vi "1) Single Group.vi"() -> ()   [LabVIEW 2020, in "VectoScratch.lvlib"]
uses:
  VectoScratch.lvlib
  Vecto/Group Info.ctl
  Vecto/Group Data Type.ctl
  Vecto/Channel Init.ctl
  Vecto/Group DBL/Group DBL.lvclass
  C:/dev/lv20CE/relink/lv-vecto/Vecto/Group/Group.lvclass
  Vecto/ChannelService/Create Group Abstract.vi
  Vecto/ChannelService/ChannelService.lvclass
  VectoConfig/VectoConfig.lvlib
  Vecto/Group Config/Group Config.lvclass
  Vecto/Group/Group.lvclass
panel:
  out "Channels":cluster{"Name":string, "Scaled":dbl}[](array[cluster])
  in  "stop":bool
  in  "Source Data":dbl[](array[slide])=[0.0, 0.0, 0.0, 0.0, 0.0] scale=0.0..10.0
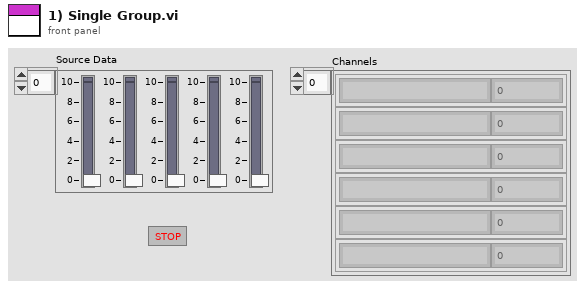
[diagram p1: front panel]
types:
  T1 = typedef "VectoConfig.lvlib/Group Data Type.ctl" = enum16{"Double", "String"}
  T2 = typedef "VectoConfig.lvlib/Group Info.ctl" = cluster{"System":string, "Cluster":string, "Node":string, "Task":string, "Name":string}
  T3 = typedef "VectoConfig.lvlib/Channel Init.ctl" = cluster{"Name":string, "Resource":string, "Unit String":string}
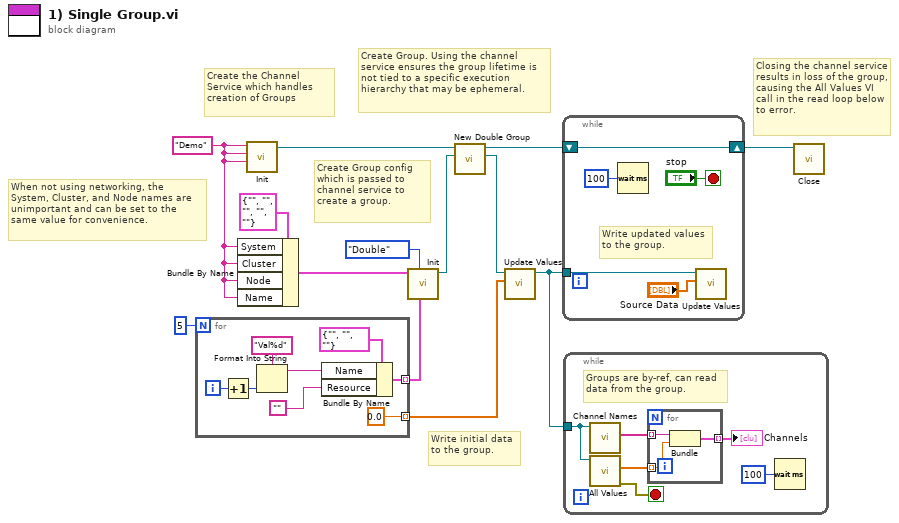
[diagram p0: block diagram]
diagram:
  w1 = "Demo" ("System")
  # "When not using networking, the System, Cluster, and Node names are unimportant and can be set to the same value for convenience."
  # "Closing the channel service results in loss of the group, causing the All Values VI call in the read loop below to error."
  # "Write initial data to the group."
  # "Create Group. Using the channel service ensures the group lifetime is not tied to a specific execution hierarchy that may be ephemeral."
  # "Create Group config which is passed to channel service to create a group."
  # "Create the Channel Service which handles creation of Groups"
  n1 = for {
    N: 5 -> [_]
    tunnel: [w15] -> w10 mode=indexing
    tunnel: [0.0] -> w7 mode=indexing
    i -> [w21]
    n2 = Increment(x=w21) -> (x+1=w20:i32)
    n3 = Format Into String(format string="Val%d", w20) -> (resulting string=w18:string)  [unwired: 2 in, 1 out]
    n4 = Bundle By Name(cluster=T3 {"Name"="", "Resource"="", "Unit String"=""} ("Channel Init"), "Name"=w18, "Resource"="") -> (w15:T3)
  }
  n5 = Bundle By Name(cluster=T2 {"System"="", "Cluster"="", "Node"="", "Task"="", "Name"=""} ("Group Info"), "System"=w1, "Cluster"=w1, "Node"=w1, "Name"=w1) -> (w11:T2)
  n6 = call "Init.vi"("Node"=w1, "Cluster"=w1, "System"=w1) -> ("ChannelService out"=w5:refnum<class "ChannelService.lvclass">)  [unwired: 7 in, 1 out]
  n7 = call "Init.vi"("Channels"=w10, "Group Data Type"=Group_Data_Type."Double", "Group Info"=w11) -> ("Group Config out"=w13:refnum<class "Group Config.lvclass">)  [unwired: 7 in, 1 out]
  n8 = call "New Double Group.vi"("Group Config"=w13, "ChannelService in"=w5) -> ("Group"=w8:refnum<class "Group DBL.lvclass">, "ChannelService out"=w2:refnum<class "ChannelService.lvclass">)  [unwired: 7 in, 1 out]
  n9 = call "Update Values.vi"("Values"=w7, "Group in"=w8) -> ("Group out"=w3:refnum<class "Group DBL.lvclass">)  [unwired: 8 in, 1 out]
  n10 = while {
    tunnel: w3 -> [w26]
    shift-right: [w22] -> w4
    shift-left: w2 -> [w22]
    stop <- "stop" stop-if-true
    # "Write updated values to the group."
    n11 = Wait (ms)(milliseconds to wait=u32 100) -> ()  [unwired: 1 out]
    n12 = call "Update Values.vi"("Values"="Source Data", "Group in"=w26) -> ()  [unwired: 8 in, 2 out]
  }
  n13 = while {
    tunnel: w3 -> [w32]
    stop <- w31 stop-if-true
    # "Groups are by-ref, can read data from the group."
    n14 = call "Channel Names.vi"("GroupAbstract in"=w32) -> ("Channel Names"=w30:string[])  [unwired: 8 in, 2 out]
    n15 = call "All Values.vi"("Group in"=w32) -> ("error out"=w31:errorcluster, "Scaled"=w29:dbl[])  [unwired: 6 in, 3 out]
    n16 = for {
      tunnel: w30 -> [w35] mode=indexing
      tunnel: w29 -> [w34] mode=indexing
      tunnel: [w33] -> w28 mode=indexing
      n17 = Bundle("Name"=w35, "Scaled"=w34) -> (w33:cluster{"Name":string, "Scaled":dbl})  [unwired: 1 in]
    }
    "Channels" <- w28
    n18 = Wait (ms)(milliseconds to wait=u32 100) -> ()  [unwired: 1 out]
  }
  n19 = call "Close.vi"("ChannelService in"=w4) -> ()  [unwired: 10 in, 1 out]
